vi "Construction_of_Subtrack(General)-2.vi"(0 "[IN] Still connected\ntracks in group":T2, 2 "[IN] Subtrack (Row of variants)":T1(array[cluster]), 3 "[IN] Index of First Pro\nblem Point Inside Track":i32, 4 "[IN] # of Track with\nFirst Problem Point":i32, 5 "error IN":errorcluster, 6 "[IN] Minimal Subtrack Len\ngth for Making Desicion":i32, 7 "[IN] Index of \nconnected dots\ninside the track":i32[](array[numeric]), 8 "[IN] Indexes for Jumps":i32[](array[numeric]), 9 "[IN] Index of connected\ntracks with problem dot":i32[](array[numeric]), 10 "[IN] Index of Initial Pro\nblem Point Inside Track":i32, 11 "[IN] # of Problem Row":i32, 12 "[IN] # of Track with\ninitial Problem Point":i32) -> (16 "[OUT] Subtracks":T1(array[cluster]), 19 "error OUT":errorcluster)   [LabVIEW 2017]
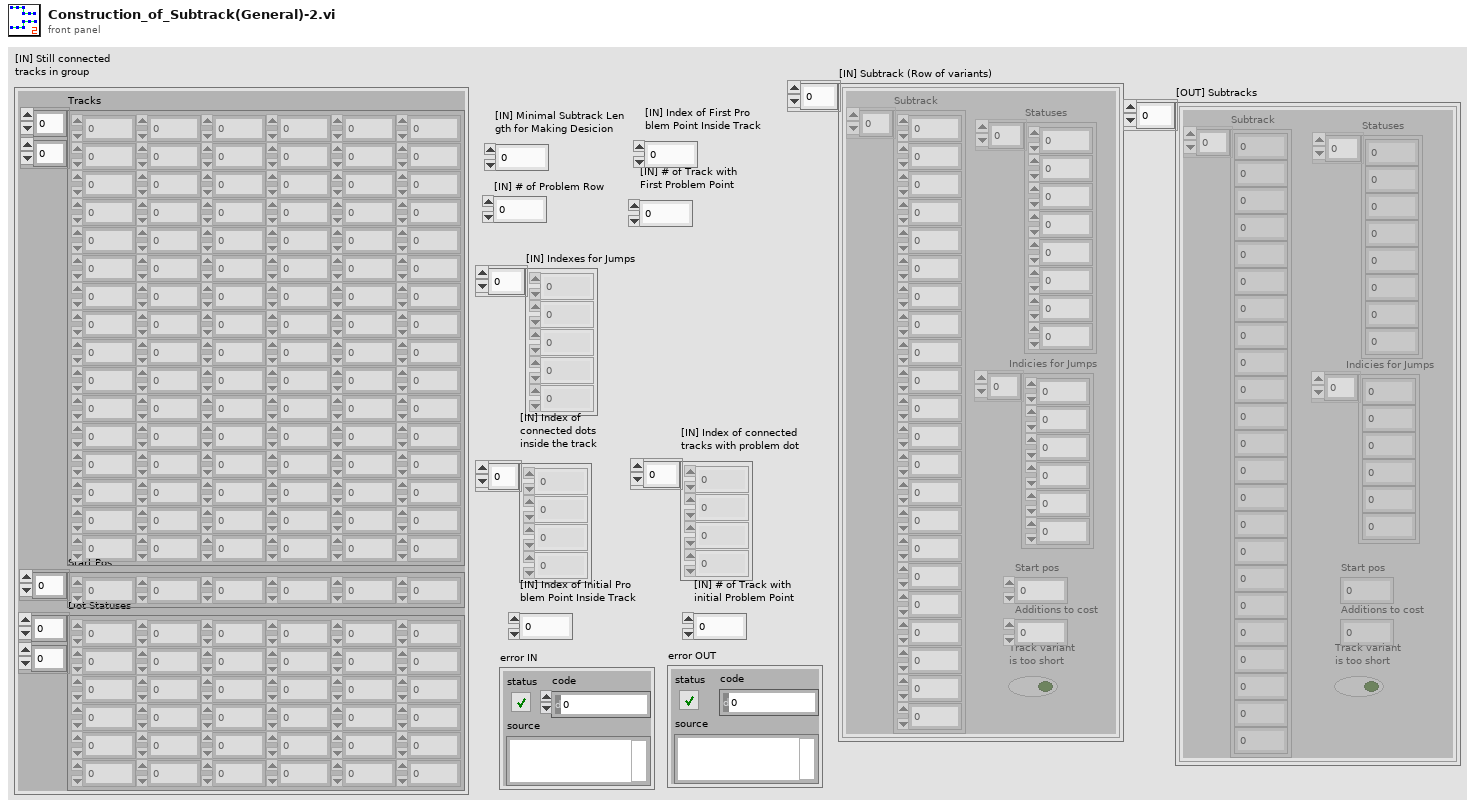
[diagram p1: front panel]
types:
  T1 = cluster{"Subtrack":dbl[], "Statuses":i16[], "Start pos":i32, "Additions to cost":i8, "Track variant \nis too short":bool, "Indicies for Jumps":i32[]}[]
  T2 = cluster{"Tracks":dbl[][], "Start Pos":i32[], "Dot Statuses":i16[][]}
  T3 = cluster{"Subtrack":dbl[], "Statuses":i16[], "Start pos":i32, "Additions to cost":i8, "Track variant \nis too short":bool, "Indicies for Jumps":i32[]}
  T4 = cluster{"Subtrack":dbl[], "Statuses":i16[], "Start pos":i32, "Additions to cost":i8, "Track variant \nis too short":bool, "Indexes for Jumps":i32[]}
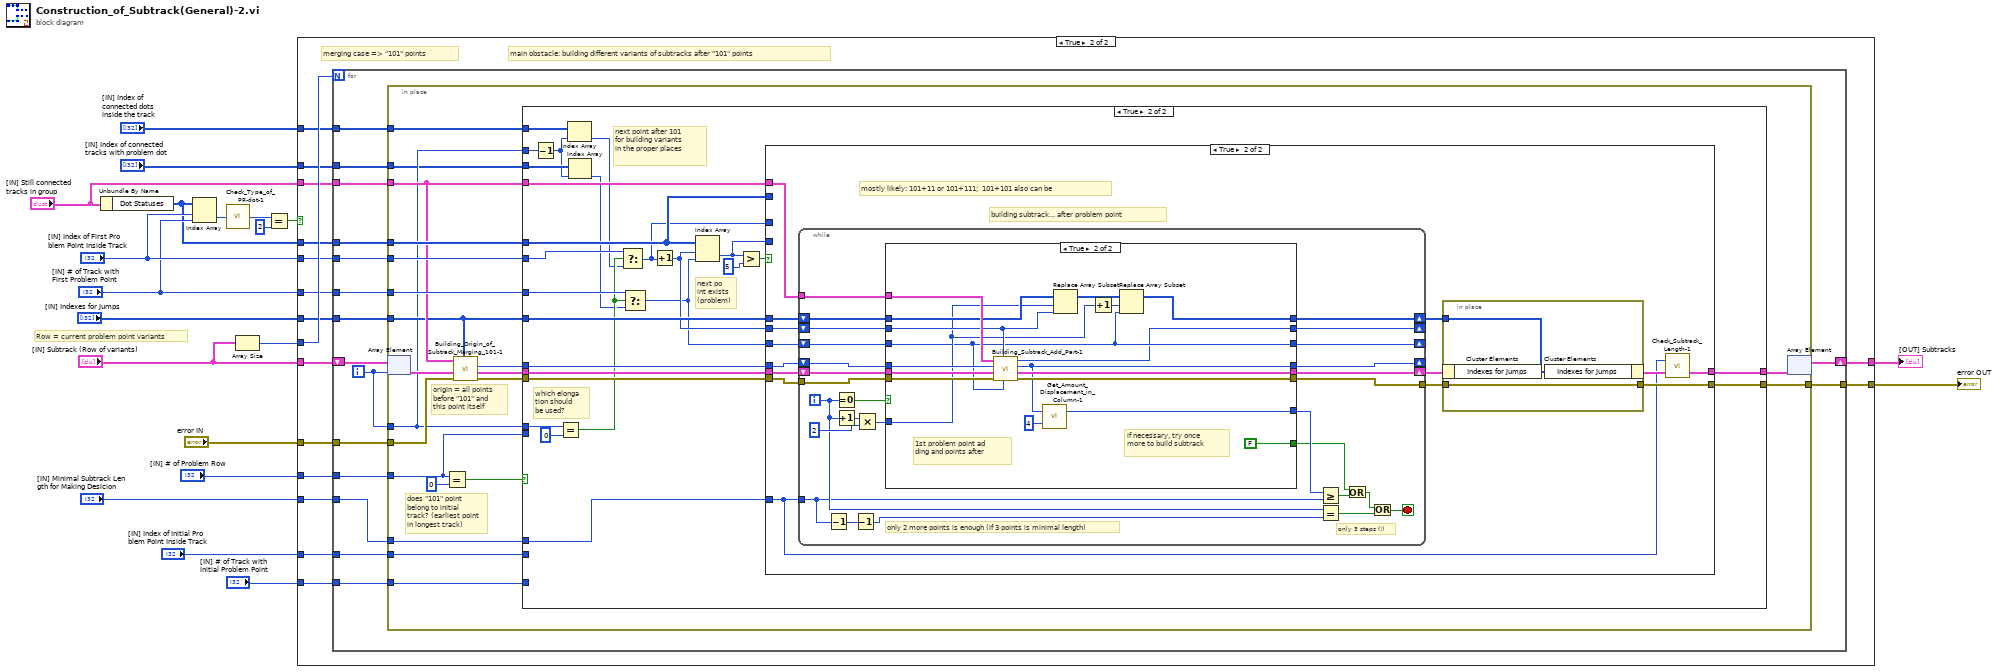
[diagram p0: block diagram]
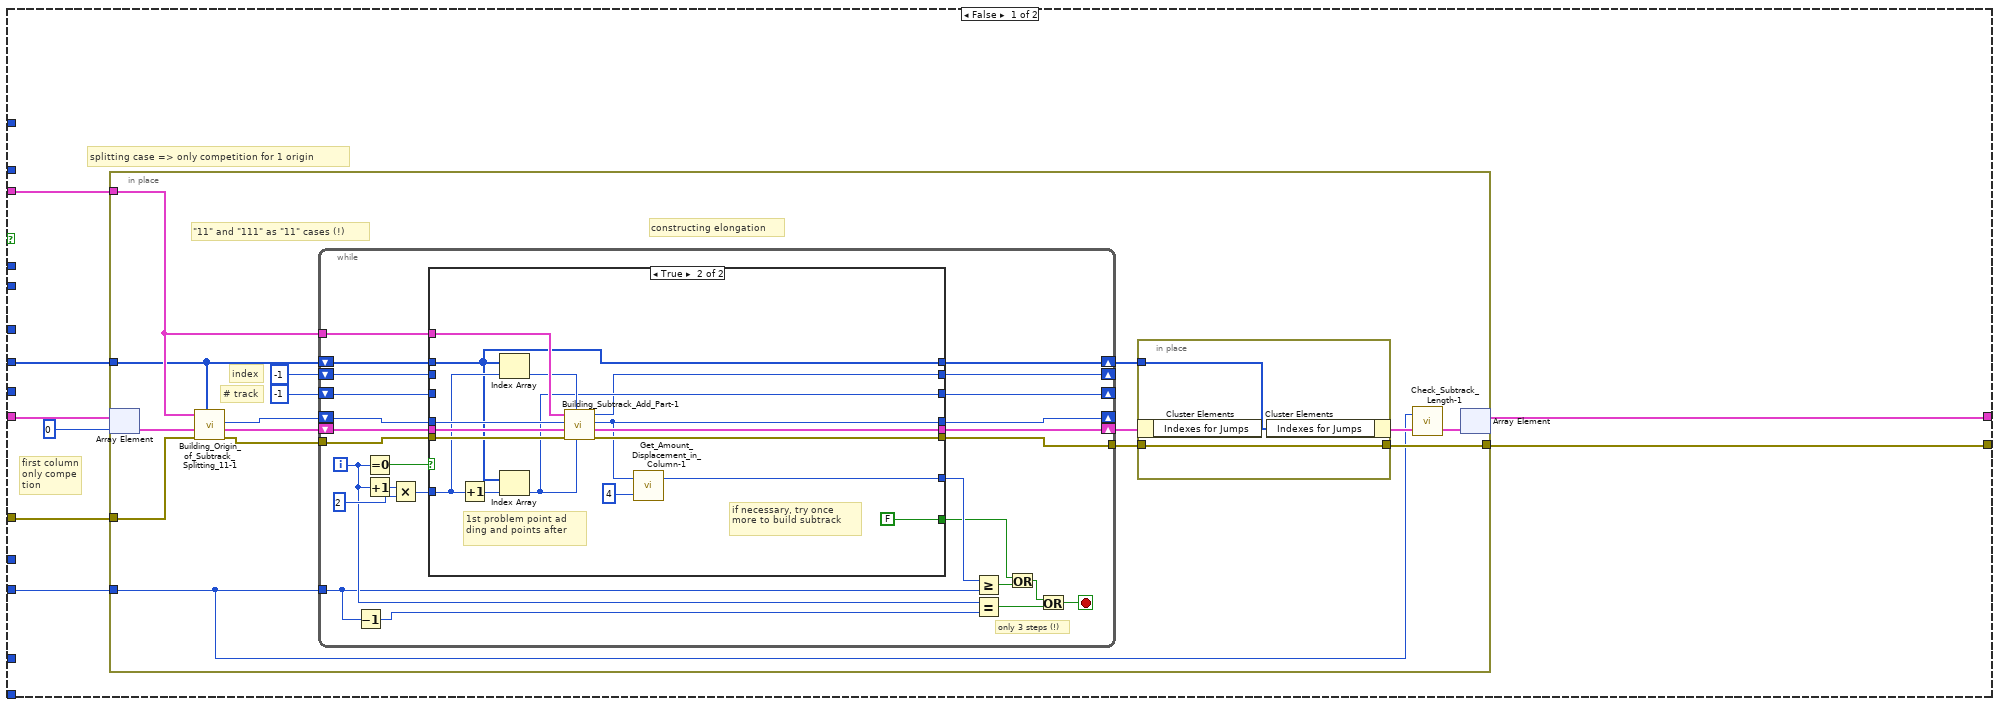
[diagram p2: hidden frame]
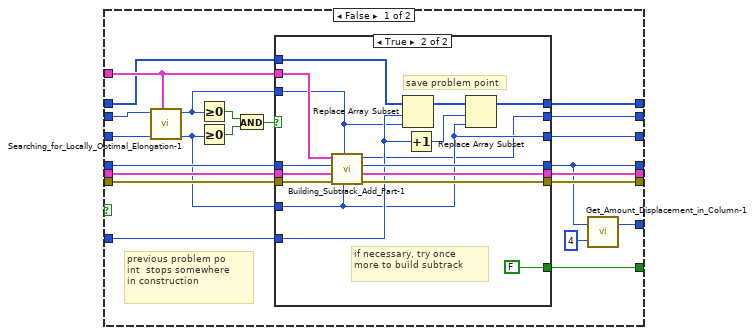
[diagram p3: hidden frame]
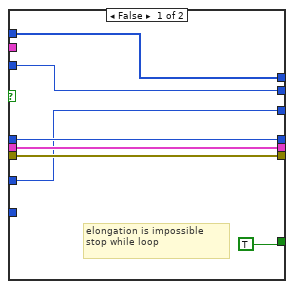
[diagram p4: hidden frame]
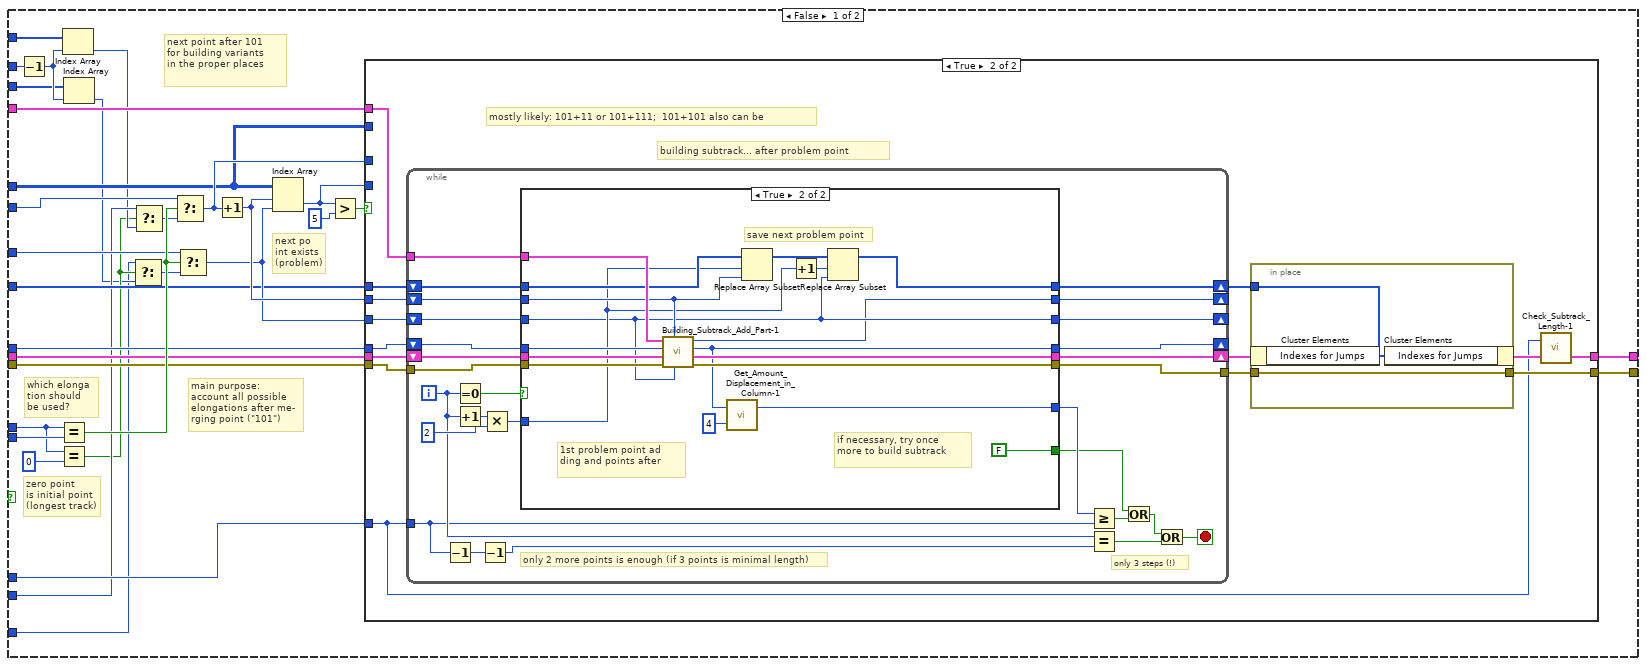
[diagram p5: hidden frame]
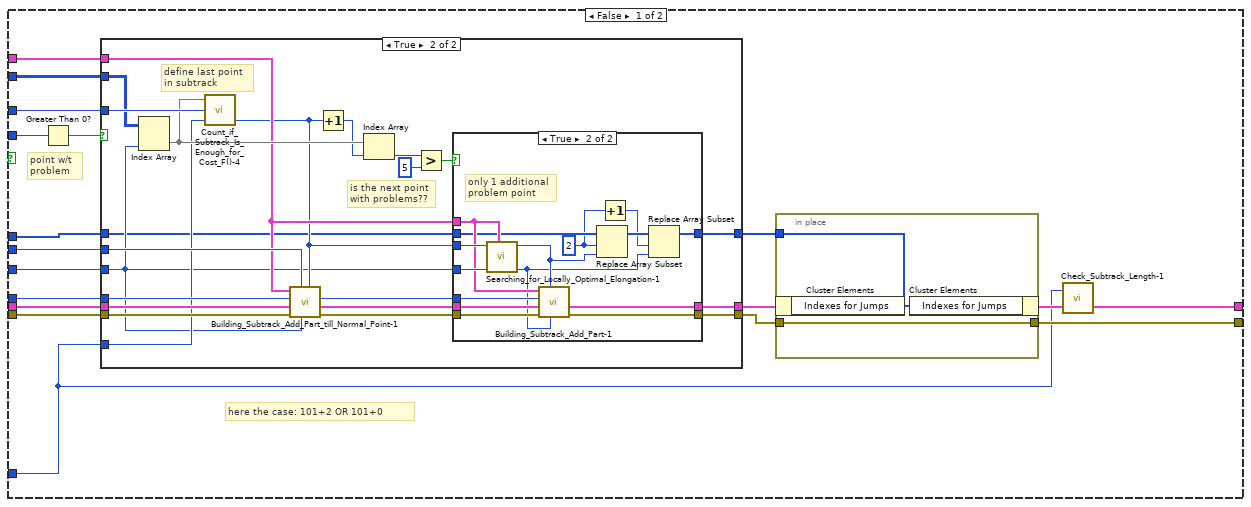
[diagram p6: hidden frame]
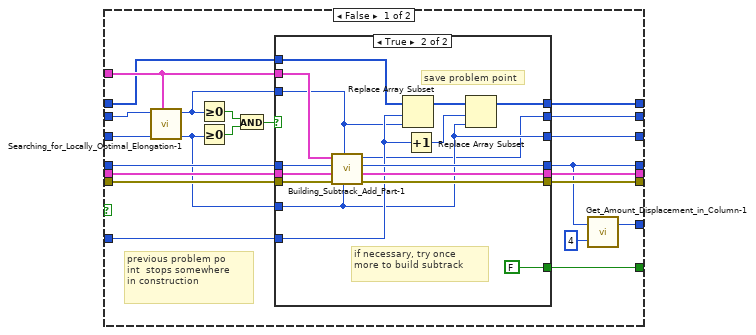
[diagram p9: hidden frame]
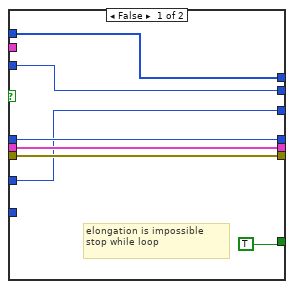
[diagram p10: hidden frame]
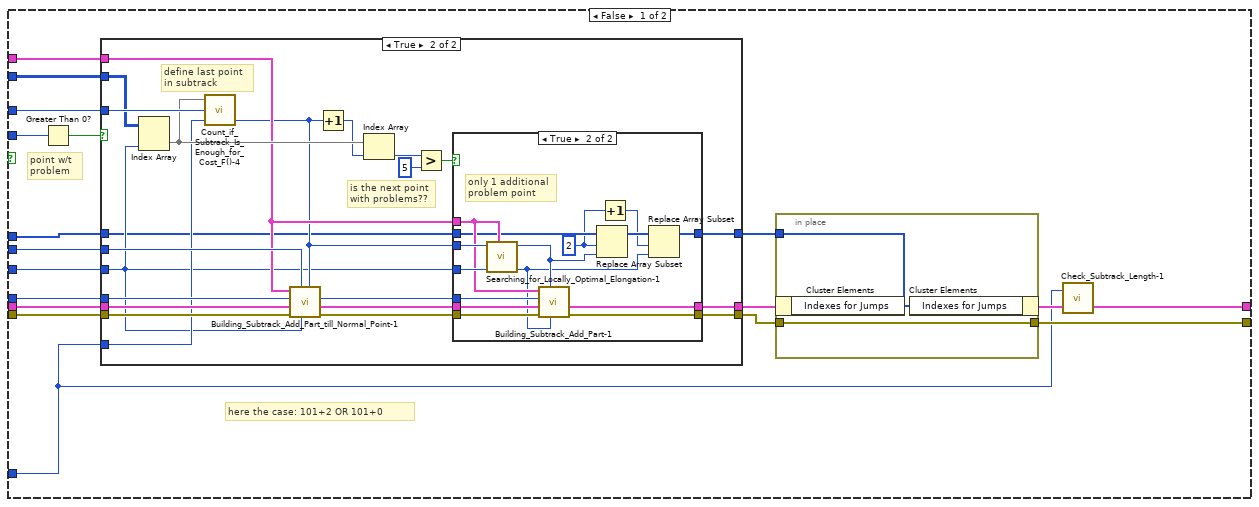
[diagram p11: hidden frame]
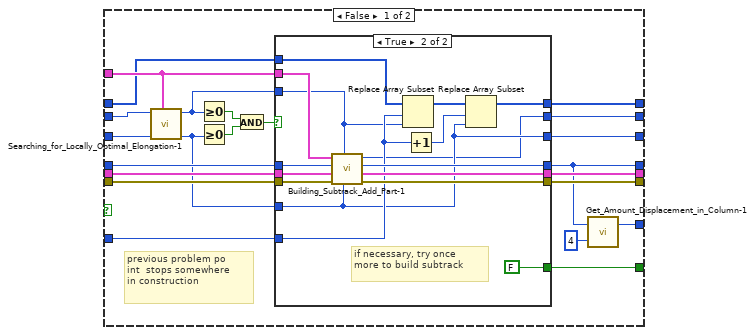
[diagram p14: hidden frame]
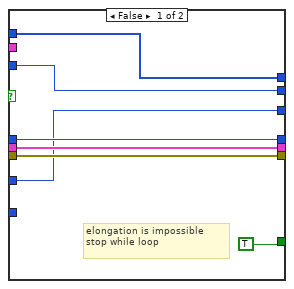
[diagram p15: hidden frame]
diagram:
  # "Row = current problem point variants"
  n1 = Unbundle By Name("[IN] Still connected\ntracks in group") -> ("Dot Statuses"=w5:i16[][])
  n2 = Index Array(array=w5, index (row)="[IN] Index of First Pro\nblem Point Inside Track", index (col)="[IN] # of Track with\nFirst Problem Point") -> (element=w20:i16)
  n3 = call "Check_Type_of_PR-dot-1.vi"("[IN] dot status"=w20) -> ("[OUT] Type of\nproblem dot"=w18:i32)
  n4 = Array Size(array="[IN] Subtrack (Row of variants)") -> (size(s)=w6:i32)
  n5 = Equal?(x=w18, y=2) -> (x = y?=w17:bool)
  n6 = case shown="True" w17 {
    tunnel: "[IN] Index of First Pro\nblem Point Inside Track" -> [_ w143]
    tunnel: "[IN] Indexes for Jumps" -> [w26 w144]
    tunnel: "[IN] Subtrack (Row of variants)" -> [w23 w149]
    tunnel: "[IN] # of Track with\nFirst Problem Point" -> [_ w142]
    tunnel: "error IN" -> [w28 w146]
    tunnel: "[IN] Still connected\ntracks in group" -> [w27 w145]
    tunnel: "[IN] Minimal Subtrack Len\ngth for Making Desicion" -> [w25 w140]
    tunnel: [w22 w138] -> w10
    tunnel: [w24 w139] -> w9
    tunnel: "[IN] # of Problem Row" -> [_ w148]
    tunnel: w6 -> [_ w147]
    tunnel: w5 -> [_ w141]
    tunnel: "[IN] Index of \nconnected dots\ninside the track" -> [_ w137]
    tunnel: "[IN] Index of connected\ntracks with problem dot" -> [_ w136]
    tunnel: "[IN] Index of Initial Pro\nblem Point Inside Track" -> [_ w135]
    tunnel: "[IN] # of Track with\ninitial Problem Point" -> [_ w134]
    frame False {
      # "first column\nonly compe\ntion"
      # "splitting case => only competition for 1 origin"
      n7 = in-place {
        in-place-border: w28 -> [w44]
        in-place-border: w27 -> [w41]
        in-place-border: w26 -> [w39]
        in-place-border: w25 -> [w29]
        in-place-border: [w32] -> w24
        # "# track"
        # "index"
        # "constructing elongation"
        # "\"11\" and \"111\" as \"11\" cases (!)"
        n8 = in-place-array #1(w23, 0) -> (w36:T3)
        n9 = call "Building_Origin_of_Subtrack_Splitting_11-1.vi"("[IN] Indexes \nfor Jumps"=w39, "error IN"=w44, "[IN] Subtrack"=w36, "[IN] Still connected\ntracks in group"=w41) -> ("error OUT"=w40:errorcluster, "[OUT] Subtrack"=w42:T4, "[OUT] Last point in subtrack"=w43:i32)  [unwired: 2 in]
        n10 = while {
          shift-right: [w55] -> _
          shift-left: w43 -> [w71]
          shift-right: [w56] -> w35
          shift-left: w42 -> [w72]
          tunnel: w41 -> [w70]
          tunnel: w40 -> [w69]
          shift-right: [w63] -> _
          shift-left: -1 -> [w60]
          shift-right: [w62] -> _
          shift-left: -1 -> [w59]
          tunnel: w29 -> [w51]
          shift-right: [w58] -> w34
          shift-left: w39 -> [w64]
          tunnel: [w57] -> w33
          i -> [w52]
          stop <- w47 stop-if-true
          # "only 3 steps (!)"
          n11 = Decrement(x=w51) -> (x-1=w50:i32)
          n12 = Equal To 0?(x=w52) -> (x = 0?=w68:bool)
          n13 = Increment(x=w52) -> (x+1=w67:i32)
          n14 = Multiply(x=w67, y=2) -> (x*y=w65:i32)
          n15 = case shown="True" w68 {
            tunnel: w72 -> [w87 w133]
            tunnel: w71 -> [w86 w132]
            tunnel: w70 -> [w81 w131]
            tunnel: w69 -> [w88 w130]
            tunnel: w65 -> [w79 w129]
            tunnel: w64 -> [w80 w119]
            tunnel: [w77 w118] -> w63
            tunnel: [w76 w125] -> w62
            tunnel: [w73 w124] -> w61
            tunnel: w60 -> [w94 _]
            tunnel: w59 -> [w93 _]
            tunnel: [w78 w119] -> w58
            tunnel: [w85 w123] -> w57
            tunnel: [w84 w122] -> w56
            tunnel: [w74 w121] -> w55
            tunnel: [w89 FALSE] -> w53
            frame False {
              # "previous problem po\nint  stops somewhere\nin construction"
              n16 = call "Searching_for_Locally_Optimal_Elongation-1.vi"("[IN] Still connected\ntracks in group"=w81, "[IN] # of Track with\nSuch Problem Point"=w93, "[IN] Index of Previous Point\n(There the search stoped)"=w94) -> ("[OUT] # of Track with\nOptimal Elongation"=w82:i32, "[OUT] Index indside track \nof Optimal Elongation"=w83:i32)  [unwired: 7 in]
              n17 = Greater Or Equal To 0?(x=w83) -> (x >= 0?=w92:bool)
              n18 = Greater Or Equal To 0?(x=w82) -> (x >= 0?=w91:bool)
              n19 = And(x=w92, y=w91) -> (x .and. y?=w90:bool)
              n20 = case shown="True" w90 {
                tunnel: [TRUE FALSE] -> w89
                tunnel: w88 -> [w99 w116]
                tunnel: w87 -> [w100 w117]
                tunnel: w86 -> [w98 w111]
                tunnel: [w99 w115] -> w85
                tunnel: [w100 w114] -> w84
                tunnel: [w98 w113] -> w74
                tunnel: w83 -> [w96 w104]
                tunnel: w82 -> [w95 w103]
                tunnel: w81 -> [_ w112]
                tunnel: w80 -> [w97 w109]
                tunnel: w79 -> [_ w108]
                tunnel: [w97 w105] -> w78
                tunnel: [w96 w102] -> w77
                tunnel: [w95 w103] -> w76
                frame False {
                  # "elongation is impossible\nstop while loop"
                }
                frame True {
                  # "save problem point"
                  # "if necessary, try once \nmore to build subtrack"
                  n21 = call "Building_Subtrack_Add_Part-1.vi"("[IN] # Track with \nProblem Point"=w103, "[IN] Index of \nProblem Point"=w104, "error IN"=w116, "[IN] Subtrack"=w117, "[IN] Last Point in Subtrack"=w111, "[IN] Still connected\ntracks in group"=w112) -> ("error OUT"=w115:errorcluster, "[OUT] Subtrack"=w114:T4, "[OUT] Last point in subtrack"=w113:i32, "[OUT] Index of Last\nStop Point in Track"=w102:i32)
                  n22 = Replace Array Subset(array=w109, new element=w104, index=w108) -> (w107:i32[])
                  n23 = Increment(x=w108) -> (x+1=w106:i32)
                  n24 = Replace Array Subset(array=w107, new element=w103, index=w106) -> (w105:i32[])
                }
              }
              n25 = call "Get_Amount_Displacement_in_Column-1.vi"("multiplier"=4, "# Rows"=w74) -> ("Displ amount"=w73:i32)  [unwired: 1 out]
            }
            frame True {
              # "if necessary, try once \nmore to build subtrack"
              # "1st problem point ad\nding and points after"
              n26 = Increment(x=w129) -> (x+1=w128:i32)
              n27 = Index Array(array=w119, index=w129) -> (element=w126:i32)
              n28 = Index Array(array=w119, index=w128) -> (element=w125:i32)
              n29 = call "Building_Subtrack_Add_Part-1.vi"("[IN] # Track with \nProblem Point"=w125, "[IN] Index of \nProblem Point"=w126, "error IN"=w130, "[IN] Subtrack"=w133, "[IN] Last Point in Subtrack"=w132, "[IN] Still connected\ntracks in group"=w131) -> ("error OUT"=w123:errorcluster, "[OUT] Subtrack"=w122:T4, "[OUT] Last point in subtrack"=w121:i32, "[OUT] Index of Last\nStop Point in Track"=w118:i32)
              n30 = call "Get_Amount_Displacement_in_Column-1.vi"("multiplier"=4, "# Rows"=w121) -> ("Displ amount"=w124:i32)  [unwired: 1 out]
            }
          }
          n31 = Greater Or Equal?(x=w61, y=w51) -> (x >= y?=w54:bool)
          n32 = Equal?(x=w52, y=w50) -> (x = y?=w49:bool)
          n33 = Or(x=w53, y=w54) -> (x .or. y?=w48:bool)
          n34 = Or(x=w48, y=w49) -> (x .or. y?=w47:bool)
        }
        n35 = in-place {
          in-place-border: w34 -> [w45]
          in-place-border: w33 -> [w46]
          in-place-border: [w46] -> w32
          n36 = in-place-cluster #2(w35) -> ()  [unwired: 1 out]
          n37 = in-place-cluster #2("Indexes for Jumps"=w45) -> (w31:T4)
        }
        n38 = call "Check_Subtrack_Length-1.vi"("[IN] Subtrack"=w31, "[IN] Minimal Sub\ntrack Length"=w29) -> ("[OUT] Subtrack"=w30:T4)  [unwired: 1 in]
        n39 = in-place-array #1(w30) -> (w22:T1)  [unwired: 1 out]
      }
    }
    frame True {
      # "main obstacle: building different variants of subtracks after \"101\" points"
      # "merging case => \"101\" points"
      n40 = for {
        N: w147 -> [_]
        shift-right: [w155] -> w138
        shift-left: w149 -> [w165]
        tunnel: w148 -> [w161]
        tunnel: w146 -> [w164]
        tunnel: w145 -> [w163]
        tunnel: w144 -> [w162]
        tunnel: w143 -> [w160]
        tunnel: w142 -> [w159]
        tunnel: w141 -> [w158]
        tunnel: w140 -> [w156]
        tunnel: [w154] -> w139
        tunnel: w137 -> [w153]
        tunnel: w136 -> [w152]
        tunnel: w135 -> [w151]
        tunnel: w134 -> [w150]
        i -> [w157]
        n41 = in-place {
          in-place-border: w164 -> [w185]
          in-place-border: w163 -> [w176]
          in-place-border: w162 -> [w174]
          in-place-border: w161 -> [w166]
          in-place-border: w160 -> [w182]
          in-place-border: w159 -> [w181]
          in-place-border: w158 -> [w180]
          in-place-border: w157 -> [w171]
          in-place-border: w156 -> [w175]
          in-place-border: [w172] -> w154
          in-place-border: w153 -> [w170]
          in-place-border: w152 -> [w169]
          in-place-border: w151 -> [w168]
          in-place-border: w150 -> [w167]
          # "does \"101\" point \nbelong to initial\ntrack? (earliest point\nin longest track)"
          # "origin = all points \nbefore \"101\" and \nthis point itself"
          n42 = in-place-array #3(w165, w157) -> (w186:T3)
          n43 = Equal?(x=w166, y=0) -> (x = y?=w183:bool)
          n44 = call "Building_Origin_of_Subtrack_Merging_101-1.vi"("[IN] Indexes \nfor Jumps"=w174, "error IN"=w185, "[IN] Subtrack"=w186, "[IN] Still connected\ntracks in group"=w176) -> ("error OUT"=w177:errorcluster, "[OUT] Subtrack"=w179:T4, "[OUT] Last point in subtrack"=w178:i32)  [unwired: 2 in]
          n45 = case shown="True" w183 {
            tunnel: w182 -> [w205 w398]
            tunnel: w181 -> [w206 w392]
            tunnel: w180 -> [w204 w411]
            tunnel: w171 -> [w195 w413]
            tunnel: w179 -> [w209 w409]
            tunnel: w178 -> [w210 w410]
            tunnel: w177 -> [w208 w408]
            tunnel: w176 -> [w203 w407]
            tunnel: w175 -> [w199 w406]
            tunnel: w174 -> [w207 w405]
            tunnel: [w198 w404] -> w173
            tunnel: [w197 w403] -> w172
            tunnel: w171 -> [w201 w396]
            tunnel: w170 -> [w200 w395]
            tunnel: w169 -> [w202 w394]
            tunnel: w168 -> [w193 _]
            tunnel: w167 -> [w188 _]
            tunnel: w166 -> [w196 _]
            frame False {
              # "zero point\nis initial point\n(longest track)"
              # "main purpose: \naccount all possible\nelongations after me-\nrging point (\"101\")"
              # "next point after 101\nfor building variants\nin the proper places"
              # "next po\nint exists\n(problem)"
              # "which elonga\ntion should \nbe used?"
              n46 = Decrement(x=w201) -> (x-1=w213:i32)
              n47 = Equal?(x=w195, y=w196) -> (x = y?=w212:bool)
              n48 = Equal?(x=w195, y=0) -> (x = y?=w190:bool)
              n49 = Index Array(array=w200, index=w213) -> (element=w191:i32)
              n50 = Index Array(array=w202, index=w213) -> (element=w189:i32)
              n51 = Select(t=w188, s=w190, f=w189) -> (s? t:f=w187:i32)
              n52 = Select(t=w193, s=w190, f=w191) -> (s? t:f=w192:i32)
              n53 = Select(t=w205, s=w212, f=w192) -> (s? t:f=w214:i32)
              n54 = Select(t=w206, s=w212, f=w187) -> (s? t:f=w211:i32)
              n55 = Increment(x=w214) -> (x+1=w218:i32)
              n56 = Index Array(array=w204, index (row)=w218, index (col)=w211) -> (element=w215:i16)
              n57 = Greater?(x=w215, y=i16 5) -> (0:w216:bool)
              n58 = case shown="True" w216 {
                tunnel: w208 -> [w228 w293]
                tunnel: w209 -> [w229 w295]
                tunnel: w210 -> [w227 w294]
                tunnel: w211 -> [w232 w292]
                tunnel: w218 -> [w230 w291]
                tunnel: w203 -> [w231 w290]
                tunnel: w199 -> [w219 w283]
                tunnel: w207 -> [w226 w289]
                tunnel: w215 -> [w236 _]
                tunnel: w214 -> [w235 _]
                tunnel: [w220 w284] -> w197
                tunnel: [w221 w282] -> w198
                tunnel: w204 -> [w233 _]
                frame False {
                  # "here the case: 101+2 OR 101+0"
                  # "point w/t \nproblem"
                  n59 = Greater Than 0?(x=w236) -> (x > 0?=w234:bool)
                  n60 = case shown="True" w234 {
                    tunnel: w235 -> [_ w263]
                    tunnel: w233 -> [_ w262]
                    tunnel: w219 -> [_ w248]
                    tunnel: w232 -> [_ w246]
                    tunnel: w231 -> [_ w250]
                    tunnel: w230 -> [_ w261]
                    tunnel: w229 -> [w241 w260]
                    tunnel: w228 -> [w240 w259]
                    tunnel: w227 -> [_ w258]
                    tunnel: [w241 w245] -> w224
                    tunnel: [w240 w244] -> w223
                    tunnel: w226 -> [w239 w243]
                    tunnel: [w239 w242] -> w222
                    frame False {
                      # "this case can be only if next point is zero"
                    }
                    frame True {
                      # "is the next point\nwith problems??"
                      # "define last point \nin subtrack"
                      n61 = Index Array(array=w262, index (col)=w246) -> (element=w257:i16[])  [unwired: 1 in]
                      n62 = call "Count_if_Subtrack_Is_Enough_for_Cost_F()-4.vi"("[IN] Minimal Subtrack Length \n(Points without problems) for\nMaking Desicion"=w248, "[IN] Index of Problem \nPoint Inside Track"=w263, "[IN] Dot Statuses in Track"=w257) -> ("[OUT] Index of Last \nPoint in Track"=w247:i32)  [unwired: 1 in, 1 out]
                      n63 = call "Building_Subtrack_Add_Part_till_Normal_Point-1.vi"("[IN] Last Normal Poi\nnt after 101 Problem"=w247, "[IN] # Track with \n101 Problem Point"=w246, "[IN] Index of \nPoint after 101"=w261, "error IN"=w259, "[IN] Subtrack"=w260, "[IN] Last Point in Subtrack"=w258, "[IN] Still connected\ntracks in group"=w250) -> ("error OUT"=w252:errorcluster, "[OUT] Subtrack"=w253:T4, "[OUT] Last point in subtrack"=w251:i32)  [unwired: 1 in]
                      n64 = Increment(x=w247) -> (x+1=w249:i32)
                      n65 = Index Array(array=w257, index=w249) -> (element=w256:i16)
                      n66 = Greater?(x=w256, y=i16 5) -> (0:w254:bool)
                      n67 = case shown="True" w254 {
                        tunnel: w253 -> [w265 w281]
                        tunnel: w252 -> [w264 w280]
                        tunnel: w251 -> [_ w279]
                        tunnel: w250 -> [_ w276]
                        tunnel: w247 -> [_ w278]
                        tunnel: w246 -> [_ w277]
                        tunnel: [w265 w275] -> w245
                        tunnel: [w264 w274] -> w244
                        tunnel: w243 -> [w266 w273]
                        tunnel: [w266 w267] -> w242
                        frame False {
                          # "only in one case\nthis point is zero"
                        }
                        frame True {
                          w270 = 2 ("index")
                          # "only 1 additional\nproblem point"
                          n68 = call "Searching_for_Locally_Optimal_Elongation-1.vi"("[IN] Still connected\ntracks in group"=w276, "[IN] # of Track with\nSuch Problem Point"=w277, "[IN] Index of Previous Point\n(There the search stoped)"=w278) -> ("[OUT] # of Track with\nOptimal Elongation"=w268:i32, "[OUT] Index indside track \nof Optimal Elongation"=w272:i32)  [unwired: 7 in]
                          n69 = call "Building_Subtrack_Add_Part-1.vi"("[IN] # Track with \nProblem Point"=w268, "[IN] Index of \nProblem Point"=w272, "error IN"=w280, "[IN] Subtrack"=w281, "[IN] Last Point in Subtrack"=w279, "[IN] Still connected\ntracks in group"=w276) -> ("error OUT"=w274:errorcluster, "[OUT] Subtrack"=w275:T4)  [unwired: 2 out]
                          n70 = Replace Array Subset(array=w273, new element=w272, index=w270) -> (w271:i32[])
                          n71 = Increment(x=w270) -> (x+1=w269:i32)
                          n72 = Replace Array Subset(array=w271, new element=w268, index=w269) -> (w267:i32[])
                        }
                      }
                    }
                  }
                  n73 = in-place {
                    in-place-border: w222 -> [w237]
                    in-place-border: w223 -> [w238]
                    in-place-border: [w238] -> w220
                    n74 = in-place-cluster #4(w224) -> ()  [unwired: 1 out]
                    n75 = in-place-cluster #4("Indexes for Jumps"=w237) -> (w225:T4)
                  }
                  n76 = call "Check_Subtrack_Length-1.vi"("[IN] Subtrack"=w225, "[IN] Minimal Sub\ntrack Length"=w219) -> ("[OUT] Subtrack"=w221:T4)  [unwired: 1 in]
                }
                frame True {
                  # "mostly likely: 101+11 or 101+111;  101+101 also can be"
                  # "building subtrack... after problem point"
                  n77 = while {
                    shift-right: [w307] -> _
                    shift-left: w294 -> [w323]
                    shift-right: [w308] -> w285
                    shift-left: w295 -> [w324]
                    tunnel: w290 -> [w322]
                    tunnel: w293 -> [w321]
                    shift-right: [w315] -> _
                    shift-left: w291 -> [w312]
                    shift-right: [w314] -> _
                    shift-left: w292 -> [w311]
                    tunnel: w283 -> [w303]
                    shift-right: [w310] -> w286
                    shift-left: w289 -> [w316]
                    tunnel: [w309] -> w287
                    i -> [w304]
                    stop <- w300 stop-if-true
                    # "only 2 more points is enough (if 3 points is minimal length)"
                    # "only 3 steps (!)"
                    n78 = Decrement(x=w303) -> (x-1=w299:i32)
                    n79 = Equal To 0?(x=w304) -> (x = 0?=w320:bool)
                    n80 = Increment(x=w304) -> (x+1=w319:i32)
                    n81 = Decrement(x=w299) -> (x-1=w298:i32)
                    n82 = Multiply(x=w319, y=2) -> (x*y=w317:i32)
                    n83 = case shown="True" w320 {
                      tunnel: w324 -> [w339 w387]
                      tunnel: w323 -> [w338 w386]
                      tunnel: w322 -> [w333 w385]
                      tunnel: w321 -> [w340 w384]
                      tunnel: w317 -> [w331 w373]
                      tunnel: w316 -> [w332 w377]
                      tunnel: [w329 w370] -> w315
                      tunnel: [w328 w371] -> w314
                      tunnel: [w325 w382] -> w313
                      tunnel: w312 -> [w346 w376]
                      tunnel: w311 -> [w345 w371]
                      tunnel: [w330 w374] -> w310
                      tunnel: [w337 w381] -> w309
                      tunnel: [w336 w380] -> w308
                      tunnel: [w326 w379] -> w307
                      tunnel: [w341 FALSE] -> w305
                      frame False {
                        # "previous problem po\nint  stops somewhere\nin construction"
                        n84 = call "Searching_for_Locally_Optimal_Elongation-1.vi"("[IN] Still connected\ntracks in group"=w333, "[IN] # of Track with\nSuch Problem Point"=w345, "[IN] Index of Previous Point\n(There the search stoped)"=w346) -> ("[OUT] # of Track with\nOptimal Elongation"=w334:i32, "[OUT] Index indside track \nof Optimal Elongation"=w335:i32)  [unwired: 7 in]
                        n85 = Greater Or Equal To 0?(x=w335) -> (x >= 0?=w344:bool)
                        n86 = Greater Or Equal To 0?(x=w334) -> (x >= 0?=w343:bool)
                        n87 = And(x=w344, y=w343) -> (x .and. y?=w342:bool)
                        n88 = case shown="True" w342 {
                          tunnel: [TRUE FALSE] -> w341
                          tunnel: w340 -> [w351 w368]
                          tunnel: w339 -> [w352 w369]
                          tunnel: w338 -> [w350 w363]
                          tunnel: [w351 w367] -> w337
                          tunnel: [w352 w366] -> w336
                          tunnel: [w350 w365] -> w326
                          tunnel: w335 -> [w348 w356]
                          tunnel: w334 -> [w347 w355]
                          tunnel: w333 -> [_ w364]
                          tunnel: w332 -> [w349 w361]
                          tunnel: w331 -> [_ w360]
                          tunnel: [w349 w357] -> w330
                          tunnel: [w348 w354] -> w329
                          tunnel: [w347 w355] -> w328
                          frame False {
                            # "elongation is impossible\nstop while loop"
                          }
                          frame True {
                            # "save problem point"
                            # "if necessary, try once \nmore to build subtrack"
                            n89 = call "Building_Subtrack_Add_Part-1.vi"("[IN] # Track with \nProblem Point"=w355, "[IN] Index of \nProblem Point"=w356, "error IN"=w368, "[IN] Subtrack"=w369, "[IN] Last Point in Subtrack"=w363, "[IN] Still connected\ntracks in group"=w364) -> ("error OUT"=w367:errorcluster, "[OUT] Subtrack"=w366:T4, "[OUT] Last point in subtrack"=w365:i32, "[OUT] Index of Last\nStop Point in Track"=w354:i32)
                            n90 = Replace Array Subset(array=w361, new element=w356, index=w360) -> (w359:i32[])
                            n91 = Increment(x=w360) -> (x+1=w358:i32)
                            n92 = Replace Array Subset(array=w359, new element=w355, index=w358) -> (w357:i32[])
                          }
                        }
                        n93 = call "Get_Amount_Displacement_in_Column-1.vi"("multiplier"=4, "# Rows"=w326) -> ("Displ amount"=w325:i32)  [unwired: 1 out]
                      }
                      frame True {
                        # "save next problem point"
                        # "if necessary, try once \nmore to build subtrack"
                        # "1st problem point ad\nding and points after"
                        n94 = call "Building_Subtrack_Add_Part-1.vi"("[IN] # Track with \nProblem Point"=w371, "[IN] Index of \nProblem Point"=w376, "error IN"=w384, "[IN] Subtrack"=w387, "[IN] Last Point in Subtrack"=w386, "[IN] Still connected\ntracks in group"=w385) -> ("error OUT"=w381:errorcluster, "[OUT] Subtrack"=w380:T4, "[OUT] Last point in subtrack"=w379:i32, "[OUT] Index of Last\nStop Point in Track"=w370:i32)
                        n95 = call "Get_Amount_Displacement_in_Column-1.vi"("multiplier"=4, "# Rows"=w379) -> ("Displ amount"=w382:i32)  [unwired: 1 out]
                        n96 = Replace Array Subset(array=w377, new element=w376, index=w373) -> (w375:i32[])
                        n97 = Increment(x=w373) -> (x+1=w372:i32)
                        n98 = Replace Array Subset(array=w375, new element=w371, index=w372) -> (w374:i32[])
                      }
                    }
                    n99 = Greater Or Equal?(x=w313, y=w303) -> (x >= y?=w306:bool)
                    n100 = Equal?(x=w304, y=w298) -> (x = y?=w302:bool)
                    n101 = Or(x=w305, y=w306) -> (x .or. y?=w301:bool)
                    n102 = Or(x=w301, y=w302) -> (x .or. y?=w300:bool)
                  }
                  n103 = in-place {
                    in-place-border: w286 -> [w296]
                    in-place-border: w287 -> [w297]
                    in-place-border: [w297] -> w284
                    n104 = in-place-cluster #5(w285) -> ()  [unwired: 1 out]
                    n105 = in-place-cluster #5("Indexes for Jumps"=w296) -> (w288:T4)
                  }
                  n106 = call "Check_Subtrack_Length-1.vi"("[IN] Subtrack"=w288, "[IN] Minimal Sub\ntrack Length"=w283) -> ("[OUT] Subtrack"=w282:T4)  [unwired: 1 in]
                }
              }
            }
            frame True {
              # "next point after 101\nfor building variants\nin the proper places"
              # "next po\nint exists\n(problem)"
              # "which elonga\ntion should \nbe used?"
              n107 = Decrement(x=w396) -> (x-1=w393:i32)
              n108 = Equal?(x=w413, y=0) -> (x = y?=w391:bool)
              n109 = Index Array(array=w395, index=w393) -> (element=w389:i32)
              n110 = Index Array(array=w394, index=w393) -> (element=w388:i32)
              n111 = Select(t=w398, s=w391, f=w389) -> (s? t:f=w397:i32)
              n112 = Select(t=w392, s=w391, f=w388) -> (s? t:f=w390:i32)
              n113 = Increment(x=w397) -> (x+1=w402:i32)
              n114 = Index Array(array=w411, index (row)=w402, index (col)=w390) -> (element=w399:i16)
              n115 = Greater?(x=w399, y=i16 5) -> (0:w400:bool)
              n116 = case shown="True" w400 {
                tunnel: w408 -> [w423 w488]
                tunnel: w409 -> [w424 w490]
                tunnel: w410 -> [w422 w489]
                tunnel: w390 -> [w427 w487]
                tunnel: w402 -> [w425 w486]
                tunnel: w407 -> [w426 w485]
                tunnel: w406 -> [w414 w478]
                tunnel: w405 -> [w421 w484]
                tunnel: w399 -> [w431 _]
                tunnel: w397 -> [w430 _]
                tunnel: [w415 w479] -> w403
                tunnel: [w416 w477] -> w404
                tunnel: w411 -> [w428 _]
                frame False {
                  # "here the case: 101+2 OR 101+0"
                  # "point w/t \nproblem"
                  n117 = Greater Than 0?(x=w431) -> (x > 0?=w429:bool)
                  n118 = case shown="True" w429 {
                    tunnel: w430 -> [_ w458]
                    tunnel: w428 -> [_ w457]
                    tunnel: w414 -> [_ w443]
                    tunnel: w427 -> [_ w441]
                    tunnel: w426 -> [_ w445]
                    tunnel: w425 -> [_ w456]
                    tunnel: w424 -> [w436 w455]
                    tunnel: w423 -> [w435 w454]
                    tunnel: w422 -> [_ w453]
                    tunnel: [w436 w440] -> w419
                    tunnel: [w435 w439] -> w418
                    tunnel: w421 -> [w434 w438]
                    tunnel: [w434 w437] -> w417
                    frame False {
                      # "this case can be only if next point is zero"
                    }
                    frame True {
                      # "is the next point\nwith problems??"
                      # "define last point \nin subtrack"
                      n119 = Index Array(array=w457, index (col)=w441) -> (element=w452:i16[])  [unwired: 1 in]
                      n120 = call "Count_if_Subtrack_Is_Enough_for_Cost_F()-4.vi"("[IN] Minimal Subtrack Length \n(Points without problems) for\nMaking Desicion"=w443, "[IN] Index of Problem \nPoint Inside Track"=w458, "[IN] Dot Statuses in Track"=w452) -> ("[OUT] Index of Last \nPoint in Track"=w442:i32)  [unwired: 1 in, 1 out]
                      n121 = call "Building_Subtrack_Add_Part_till_Normal_Point-1.vi"("[IN] Last Normal Poi\nnt after 101 Problem"=w442, "[IN] # Track with \n101 Problem Point"=w441, "[IN] Index of \nPoint after 101"=w456, "error IN"=w454, "[IN] Subtrack"=w455, "[IN] Last Point in Subtrack"=w453, "[IN] Still connected\ntracks in group"=w445) -> ("error OUT"=w447:errorcluster, "[OUT] Subtrack"=w448:T4, "[OUT] Last point in subtrack"=w446:i32)  [unwired: 1 in]
                      n122 = Increment(x=w442) -> (x+1=w444:i32)
                      n123 = Index Array(array=w452, index=w444) -> (element=w451:i16)
                      n124 = Greater?(x=w451, y=i16 5) -> (0:w449:bool)
                      n125 = case shown="True" w449 {
                        tunnel: w448 -> [w460 w476]
                        tunnel: w447 -> [w459 w475]
                        tunnel: w446 -> [_ w474]
                        tunnel: w445 -> [_ w471]
                        tunnel: w442 -> [_ w473]
                        tunnel: w441 -> [_ w472]
                        tunnel: [w460 w470] -> w440
                        tunnel: [w459 w469] -> w439
                        tunnel: w438 -> [w461 w468]
                        tunnel: [w461 w462] -> w437
                        frame False {
                          # "only in one case\nthis point is zero"
                        }
                        frame True {
                          w465 = 2 ("index")
                          # "only 1 additional\nproblem point"
                          n126 = call "Searching_for_Locally_Optimal_Elongation-1.vi"("[IN] Still connected\ntracks in group"=w471, "[IN] # of Track with\nSuch Problem Point"=w472, "[IN] Index of Previous Point\n(There the search stoped)"=w473) -> ("[OUT] # of Track with\nOptimal Elongation"=w463:i32, "[OUT] Index indside track \nof Optimal Elongation"=w467:i32)  [unwired: 7 in]
                          n127 = call "Building_Subtrack_Add_Part-1.vi"("[IN] # Track with \nProblem Point"=w463, "[IN] Index of \nProblem Point"=w467, "error IN"=w475, "[IN] Subtrack"=w476, "[IN] Last Point in Subtrack"=w474, "[IN] Still connected\ntracks in group"=w471) -> ("error OUT"=w469:errorcluster, "[OUT] Subtrack"=w470:T4)  [unwired: 2 out]
                          n128 = Replace Array Subset(array=w468, new element=w467, index=w465) -> (w466:i32[])
                          n129 = Increment(x=w465) -> (x+1=w464:i32)
                          n130 = Replace Array Subset(array=w466, new element=w463, index=w464) -> (w462:i32[])
                        }
                      }
                    }
                  }
                  n131 = in-place {
                    in-place-border: w417 -> [w432]
                    in-place-border: w418 -> [w433]
                    in-place-border: [w433] -> w415
                    n132 = in-place-cluster #6(w419) -> ()  [unwired: 1 out]
                    n133 = in-place-cluster #6("Indexes for Jumps"=w432) -> (w420:T4)
                  }
                  n134 = call "Check_Subtrack_Length-1.vi"("[IN] Subtrack"=w420, "[IN] Minimal Sub\ntrack Length"=w414) -> ("[OUT] Subtrack"=w416:T4)  [unwired: 1 in]
                }
                frame True {
                  # "mostly likely: 101+11 or 101+111;  101+101 also can be"
                  # "building subtrack... after problem point"
                  n135 = while {
                    shift-right: [w502] -> _
                    shift-left: w489 -> [w518]
                    shift-right: [w503] -> w480
                    shift-left: w490 -> [w519]
                    tunnel: w485 -> [w517]
                    tunnel: w488 -> [w516]
                    shift-right: [w510] -> _
                    shift-left: w486 -> [w507]
                    shift-right: [w509] -> _
                    shift-left: w487 -> [w506]
                    tunnel: w478 -> [w498]
                    shift-right: [w505] -> w481
                    shift-left: w484 -> [w511]
                    tunnel: [w504] -> w482
                    i -> [w499]
                    stop <- w495 stop-if-true
                    # "only 2 more points is enough (if 3 points is minimal length)"
                    # "only 3 steps (!)"
                    n136 = Decrement(x=w498) -> (x-1=w494:i32)
                    n137 = Equal To 0?(x=w499) -> (x = 0?=w515:bool)
                    n138 = Increment(x=w499) -> (x+1=w514:i32)
                    n139 = Decrement(x=w494) -> (x-1=w493:i32)
                    n140 = Multiply(x=w514, y=2) -> (x*y=w512:i32)
                    n141 = case shown="True" w515 {
                      tunnel: w519 -> [w534 w582]
                      tunnel: w518 -> [w533 w581]
                      tunnel: w517 -> [w528 w580]
                      tunnel: w516 -> [w535 w579]
                      tunnel: w512 -> [w526 w568]
                      tunnel: w511 -> [w527 w572]
                      tunnel: [w524 w565] -> w510
                      tunnel: [w523 w566] -> w509
                      tunnel: [w520 w577] -> w508
                      tunnel: w507 -> [w541 w571]
                      tunnel: w506 -> [w540 w566]
                      tunnel: [w525 w569] -> w505
                      tunnel: [w532 w576] -> w504
                      tunnel: [w531 w575] -> w503
                      tunnel: [w521 w574] -> w502
                      tunnel: [w536 FALSE] -> w500
                      frame False {
                        # "previous problem po\nint  stops somewhere\nin construction"
                        n142 = call "Searching_for_Locally_Optimal_Elongation-1.vi"("[IN] Still connected\ntracks in group"=w528, "[IN] # of Track with\nSuch Problem Point"=w540, "[IN] Index of Previous Point\n(There the search stoped)"=w541) -> ("[OUT] # of Track with\nOptimal Elongation"=w529:i32, "[OUT] Index indside track \nof Optimal Elongation"=w530:i32)  [unwired: 7 in]
                        n143 = Greater Or Equal To 0?(x=w530) -> (x >= 0?=w539:bool)
                        n144 = Greater Or Equal To 0?(x=w529) -> (x >= 0?=w538:bool)
                        n145 = And(x=w539, y=w538) -> (x .and. y?=w537:bool)
                        n146 = case shown="True" w537 {
                          tunnel: [TRUE FALSE] -> w536
                          tunnel: w535 -> [w546 w563]
                          tunnel: w534 -> [w547 w564]
                          tunnel: w533 -> [w545 w558]
                          tunnel: [w546 w562] -> w532
                          tunnel: [w547 w561] -> w531
                          tunnel: [w545 w560] -> w521
                          tunnel: w530 -> [w543 w551]
                          tunnel: w529 -> [w542 w550]
                          tunnel: w528 -> [_ w559]
                          tunnel: w527 -> [w544 w556]
                          tunnel: w526 -> [_ w555]
                          tunnel: [w544 w552] -> w525
                          tunnel: [w543 w549] -> w524
                          tunnel: [w542 w550] -> w523
                          frame False {
                            # "elongation is impossible\nstop while loop"
                          }
                          frame True {
                            # "if necessary, try once \nmore to build subtrack"
                            n147 = call "Building_Subtrack_Add_Part-1.vi"("[IN] # Track with \nProblem Point"=w550, "[IN] Index of \nProblem Point"=w551, "error IN"=w563, "[IN] Subtrack"=w564, "[IN] Last Point in Subtrack"=w558, "[IN] Still connected\ntracks in group"=w559) -> ("error OUT"=w562:errorcluster, "[OUT] Subtrack"=w561:T4, "[OUT] Last point in subtrack"=w560:i32, "[OUT] Index of Last\nStop Point in Track"=w549:i32)
                            n148 = Replace Array Subset(array=w556, new element=w551, index=w555) -> (w554:i32[])
                            n149 = Increment(x=w555) -> (x+1=w553:i32)
                            n150 = Replace Array Subset(array=w554, new element=w550, index=w553) -> (w552:i32[])
                          }
                        }
                        n151 = call "Get_Amount_Displacement_in_Column-1.vi"("multiplier"=4, "# Rows"=w521) -> ("Displ amount"=w520:i32)  [unwired: 1 out]
                      }
                      frame True {
                        # "if necessary, try once \nmore to build subtrack"
                        # "1st problem point ad\nding and points after"
                        n152 = call "Building_Subtrack_Add_Part-1.vi"("[IN] # Track with \nProblem Point"=w566, "[IN] Index of \nProblem Point"=w571, "error IN"=w579, "[IN] Subtrack"=w582, "[IN] Last Point in Subtrack"=w581, "[IN] Still connected\ntracks in group"=w580) -> ("error OUT"=w576:errorcluster, "[OUT] Subtrack"=w575:T4, "[OUT] Last point in subtrack"=w574:i32, "[OUT] Index of Last\nStop Point in Track"=w565:i32)
                        n153 = call "Get_Amount_Displacement_in_Column-1.vi"("multiplier"=4, "# Rows"=w574) -> ("Displ amount"=w577:i32)  [unwired: 1 out]
                        n154 = Replace Array Subset(array=w572, new element=w571, index=w568) -> (w570:i32[])
                        n155 = Increment(x=w568) -> (x+1=w567:i32)
                        n156 = Replace Array Subset(array=w570, new element=w566, index=w567) -> (w569:i32[])
                      }
                    }
                    n157 = Greater Or Equal?(x=w508, y=w498) -> (x >= y?=w501:bool)
                    n158 = Equal?(x=w499, y=w493) -> (x = y?=w497:bool)
                    n159 = Or(x=w500, y=w501) -> (x .or. y?=w496:bool)
                    n160 = Or(x=w496, y=w497) -> (x .or. y?=w495:bool)
                  }
                  n161 = in-place {
                    in-place-border: w481 -> [w491]
                    in-place-border: w482 -> [w492]
                    in-place-border: [w492] -> w479
                    n162 = in-place-cluster #7(w480) -> ()  [unwired: 1 out]
                    n163 = in-place-cluster #7("Indexes for Jumps"=w491) -> (w483:T4)
                  }
                  n164 = call "Check_Subtrack_Length-1.vi"("[IN] Subtrack"=w483, "[IN] Minimal Sub\ntrack Length"=w478) -> ("[OUT] Subtrack"=w477:T4)  [unwired: 1 in]
                }
              }
            }
          }
          n165 = in-place-array #3(w173) -> (w155:T1)  [unwired: 1 out]
        }
      }
    }
  }
  "error OUT" <- w9
  "[OUT] Subtracks" <- w10
